vi "main.vi"() -> ()   [LabVIEW 2018]
uses:
  <vilib>/Instr/_visa.llb/VISA Configure Serial Port (Instr).vi
panel:
  in  "baud rate":u64(ring) items=["2400"=2400, "4800"=4800, "9600"=9600, "14400"=14400, "19200"=19200, "38400"=38400, "43000"=43000, "57600"=57600, "76800"=76800, "115200"=115200]
  in  "write buffer":string
  in  "send":bool
  out "read buffer":string
  out "serial_state":bool
  in  "serial":refnum<visa-resource-name> caption="serial_select"
  in  "serial_open":bool
  in  "Exit":bool
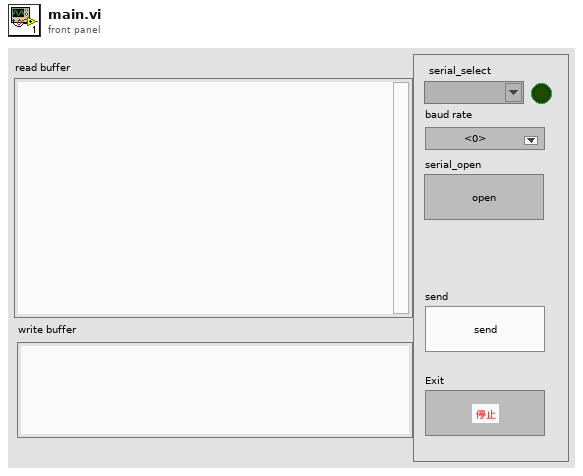
[diagram p1: front panel]
types:
  T1 = typedef "状态机.ctl" = enum16{"Init", "Wait", "GetData", "Exit"}
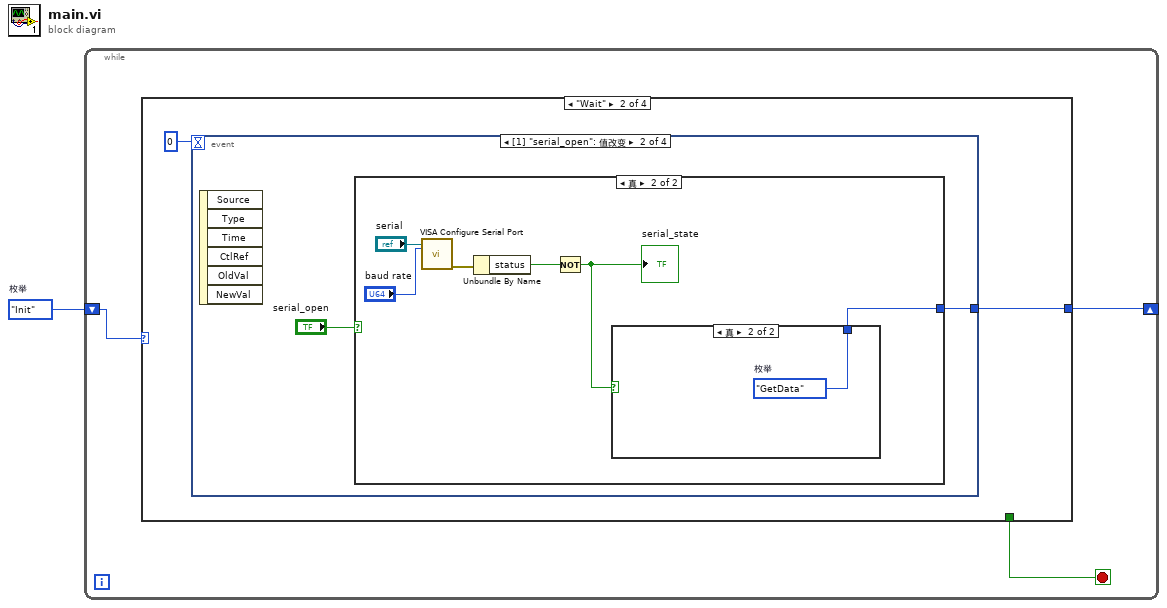
[diagram p0: block diagram]
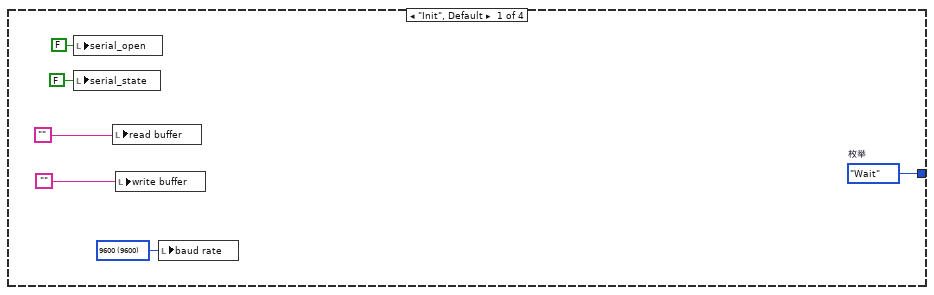
[diagram p2: hidden frame]
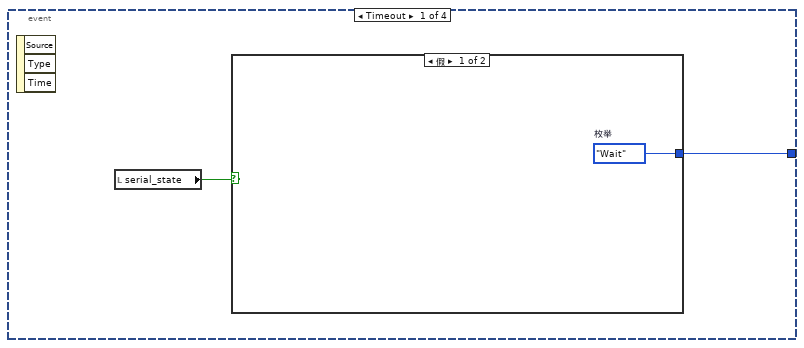
[diagram p3: hidden frame]
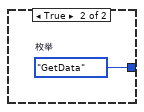
[diagram p4: hidden frame]
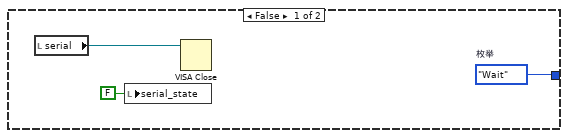
[diagram p5: hidden frame]
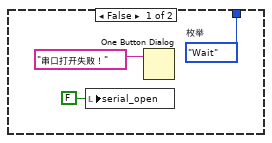
[diagram p6: hidden frame]
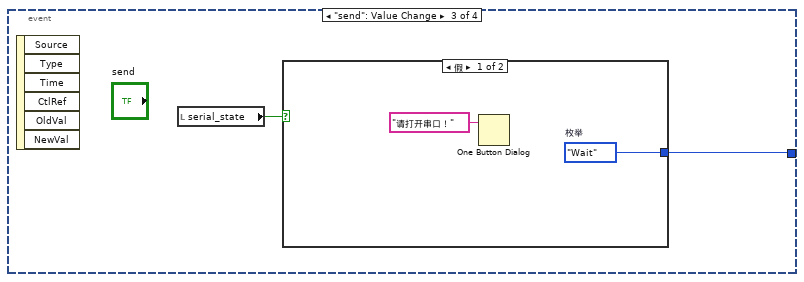
[diagram p7: hidden frame]
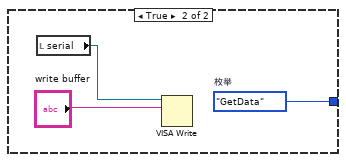
[diagram p8: hidden frame]
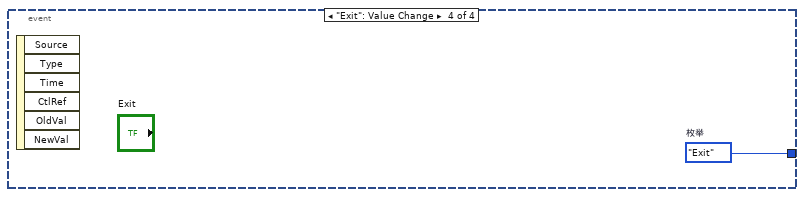
[diagram p9: hidden frame]
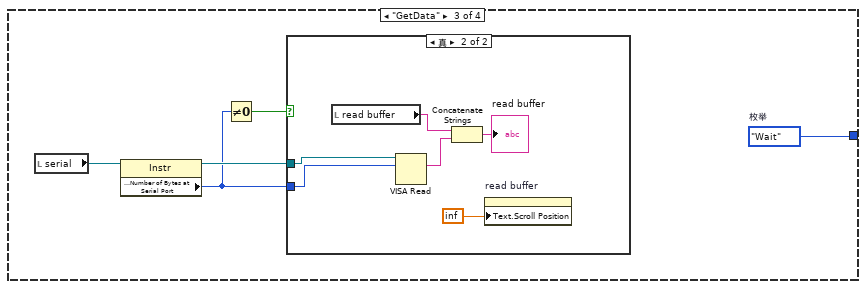
[diagram p10: hidden frame]
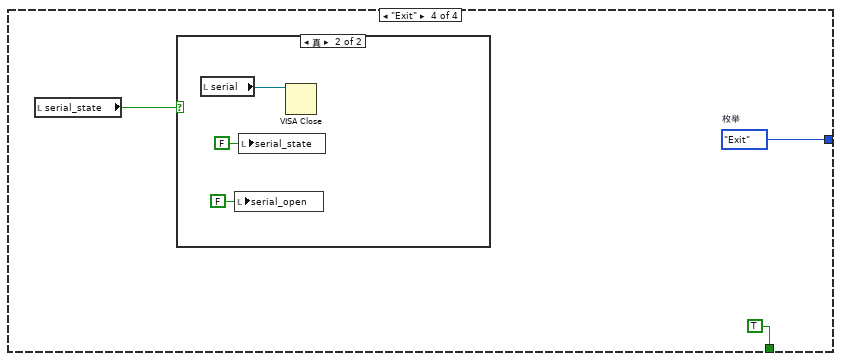
[diagram p12: hidden frame]
diagram:
  w1 = 状态机."Init"  # 枚举
  n1 = while {
    shift-right: [w3] -> _
    shift-left: w1 -> [w4]
    stop <- w2 stop-if-true
    n2 = case shown="\"Wait\"" w4 {
      tunnel: [w8 w11 w44 w53] -> w3
      tunnel: [_ _ _ TRUE] -> w2
      frame "Init", Default {
        w5 = u64 9600 items=["2400"=2400, "4800"=4800, "9600"=9600, "14400"=14400, "19200"=19200, "38400"=38400, "43000"=43000, "57600"=57600, "76800"=76800, "115200"=115200] ("baud rate")
        w8 = 状态机."Wait"  # 枚举
        n3 = local write "serial_open"(FALSE ("serial_open")) -> ()
        n4 = local write "serial_state"(FALSE ("serial_state")) -> ()
        n5 = local write "read buffer"("") -> ()
        n6 = local write "write buffer"("") -> ()
        n7 = local write "baud rate"(w5) -> ()
      }
      frame "Wait" {
        n8 = event shown="[1] \"serial_open\": 值改变" {
          selector: _ -> [_ _ _ _]
          dyn-events: _ -> [_ _ _ _]
          timeout: 0 -> [_ _ _ _]
          tunnel: [w13 w17 w32 w39] -> w11
          event Timeout {
            n9 = event-data() -> ()  [unwired: 1 in, 3 out]
            n10 = local read "serial_state"() -> (w14:bool)
            n11 = case shown="假" w14 {
              tunnel: [w15 w16] -> w13
              frame False {
                w15 = 状态机."Wait"  # 枚举
              }
              frame True {
                w16 = 状态机."GetData"  # 枚举
              }
            }
          }
          event "serial_open": Value Change {
            n12 = event-data() -> ()  [unwired: 1 in, 6 out]
            n13 = case shown="真" "serial_open" {
              tunnel: [w19 w23] -> w17
              frame False {
                w19 = 状态机."Wait"  # 枚举
                n14 = local read "serial"() -> (w21:refnum<visa-resource-name>)
                n15 = local write "serial_state"(FALSE ("serial_state")) -> ()
                n16 = VISA Close(VISA resource name=w21) -> ()  [unwired: 1 in, 1 out]
              }
              frame True {
                n17 = call-poly "VISA Configure Serial Port"("VISA resource name"="serial", "baud rate (9600)"="baud rate") -> ("error out"=w26:errorcluster)  [unwired: 12 in, 1 out]
                n18 = Unbundle By Name(w26) -> ("status"=w25:bool)
                n19 = Not(x=w25) -> (.not. x?=w24:bool)
                "serial_state" <- w24
                n20 = case shown="真" w24 {
                  tunnel: [w28 w31] -> w23
                  frame False {
                    w28 = 状态机."Wait"  # 枚举
                    n21 = local write "serial_open"(FALSE ("serial_open")) -> ()
                    n22 = One Button Dialog(message="串口打开失败！" ("消息")) -> ()  [unwired: 1 in, 1 out]
                  }
                  frame True {
                    w31 = 状态机."GetData"  # 枚举
                  }
                }
              }
            }
          }
          event "send": Value Change {
            n23 = event-data() -> ()  [unwired: 1 in, 6 out]
            n24 = local read "serial_state"() -> (w33:bool)
            n25 = case shown="假" w33 {
              tunnel: [w34 w36] -> w32
              frame False {
                w34 = 状态机."Wait"  # 枚举
                n26 = One Button Dialog(message="请打开串口！" ("消息")) -> ()  [unwired: 1 in, 1 out]
              }
              frame True {
                w36 = 状态机."GetData"  # 枚举
                n27 = local read "serial"() -> (w37:refnum<visa-resource-name>)
                n28 = VISA Write(VISA resource name=w37, write buffer="write buffer") -> ()  [unwired: 1 in, 3 out]
              }
            }
          }
          event "Exit": Value Change {
            w39 = 状态机."Exit"  # 枚举
            n29 = event-data() -> ()  [unwired: 1 in, 6 out]
          }
        }
      }
      frame "GetData" {
        w44 = 状态机."Wait"  # 枚举
        n30 = local read "serial"() -> (w40:refnum<visa-resource-name>)
        n31 = property class="Instr"(reference=w40) -> (reference out=w43:refnum<visa-resource-name>, "Serial Settings:Number of Bytes at Serial Port"=w42:u32)  [unwired: 1 in, 1 out]
        n32 = Not Equal To 0?(x=w42) -> (x != 0?=w41:bool)
        n33 = case shown="真" w41 {
          tunnel: w43 -> [_ w47]
          tunnel: w42 -> [_ w46]
          frame False {
          }
          frame True {
            n34 = local read "read buffer"() -> (w49:string)
            n35 = VISA Read(VISA resource name=w47, byte count=w46) -> (read buffer=w48:string)  [unwired: 1 in, 3 out]
            n36 = Concatenate Strings(w49, w48) -> (→"read buffer":string)
            n37 = property on="read buffer" class="Str"("Text.Scroll Position"=inf) -> ()  [unwired: 2 in, 2 out]
          }
        }
      }
      frame "Exit" {
        w53 = 状态机."Exit"  # 枚举
        n38 = local read "serial_state"() -> (w51:bool)
        n39 = case shown="真" w51 {
          frame False {
          }
          frame True {
            n40 = local read "serial"() -> (w56:refnum<visa-resource-name>)
            n41 = local write "serial_open"(FALSE ("serial_open")) -> ()
            n42 = local write "serial_state"(FALSE ("serial_state")) -> ()
            n43 = VISA Close(VISA resource name=w56) -> ()  [unwired: 1 in, 1 out]
          }
        }
      }
    }
  }
